vi "start.vi"(8 "error in (no error)":errorcluster, 11 "Application in":refnum<class "Application.lvclass">) -> (0 "error out":errorcluster, 3 "Application out":refnum<class "Application.lvclass">)   [LabVIEW 2013, in "Application.lvlib" / "Application.lvclass"]
uses:
  <userlib>/Common/Component/Application/Application/Application.lvclass
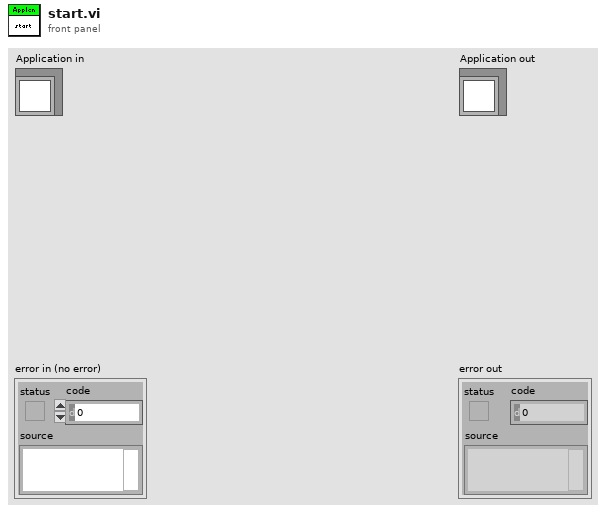
[diagram p1: front panel]
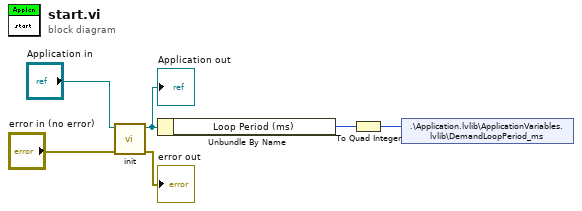
[diagram p0: block diagram]
diagram:
  n1 = call-dynamic "init.vi"("error in (no error)"="error in (no error)", "Application in"="Application in") -> ("error out"=→"error out":errorcluster, "Application out"=w1:refnum<class "Application.lvclass">)  [unwired: 8 in]
  "Application out" <- w1
  n2 = Unbundle By Name(w1) -> ("Loop Period (ms)"=w3:u16)
  n3 = To Quad Integer(1:w3) -> (0:w2:i64)
  n4 = shared-variable ".\\Application.lvlib\\ApplicationVariables.lvlib\\DemandLoopPeriod_ms"(w2) -> ()  [unwired: 1 in, 1 out]
